vi "GreaterThan.vi"(8 "error in (no error)":errorcluster, 10 "dvotTTPathPoint in 2":refnum<class "dvotTTPathPoint.lvclass">, 11 "dvotTTPathPoint in 1":refnum<class "dvotTTPathPoint.lvclass">) -> (0 "error out":errorcluster, 1 "point 1 > point 2?":bool, 2 "dvotTTPathPoint out 2":refnum<class "dvotTTPathPoint.lvclass">, 3 "dvotTTPathPoint out 1":refnum<class "dvotTTPathPoint.lvclass">)   [LabVIEW 2012, in "dvotTTPathPoint.lvclass"]
uses:
  dvotTTPathPoint.lvclass
  dvotTTPathPoint.lvclass/dvotTTPathPoint.ctl
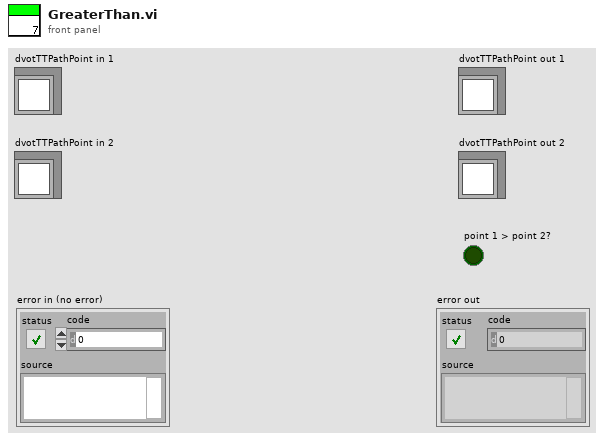
[diagram p1: front panel]
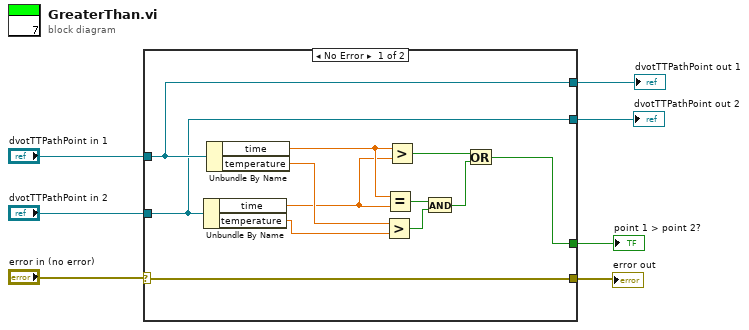
[diagram p0: block diagram]
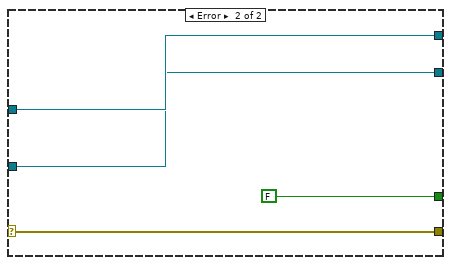
[diagram p2: hidden frame]
diagram:
  n1 = case shown="No Error" "error in (no error)" {
    selector: "error in (no error)" -> [w19 w21]
    tunnel: [w19 w21] -> w6
    tunnel: "dvotTTPathPoint in 1" -> [w18 w23]
    tunnel: "dvotTTPathPoint in 2" -> [w17 w22]
    tunnel: [w18 w23] -> w3
    tunnel: [w17 w22] -> w2
    tunnel: [w8 FALSE ("greaterThan?")] -> w1
    frame No Error {
      n2 = Unbundle By Name(w17) -> ("time"=w10:dbl, "temperature"=w12:dbl)
      n3 = Unbundle By Name(w18) -> ("time"=w11:dbl, "temperature"=w13:dbl)
      n4 = Greater?(x=w13, y=w12) -> (0:w14:bool)
      n5 = Equal?(x=w11, y=w10) -> (x = y?=w15:bool)
      n6 = Greater?(x=w11, y=w10) -> (0:w16:bool)
      n7 = And(x=w15, y=w14) -> (x .and. y?=w9:bool)
      n8 = Or(x=w16, y=w9) -> (x .or. y?=w8:bool)
    }
    frame Error {
    }
  }
  "dvotTTPathPoint out 1" <- w3
  "dvotTTPathPoint out 2" <- w2
  "point 1 > point 2?" <- w1
  "error out" <- w6
